vi "Forward by Address.vi"(6 "Message Priority (Normal)":T1=enum."Normal", 8 "error in (no error)":errorcluster, 9 "Message":refnum<class "Message.lvclass">, 10 "Target Enqueuer ID":string, 11 "Publisher in":refnum<class "Publisher.lvclass">) -> (0 "error out":errorcluster, 1 "Message forwarded?":bool, 3 "Publisher out":refnum<class "Publisher.lvclass">)   [LabVIEW 2020, in "Publisher.lvlib" / "Publisher.lvclass"]
doc: "Send 'Message' to the actor with 'Target Enqueuer ID'."
uses:
  Publisher.lvclass
  PPL/HDH.Actor Framework.Core.Actor.lvlibp/1abvi3w/vi.lib/ActorFramework/Message Enqueuer/Message Priority.ctl
  PPL/HDH.Actor Framework.Core.Actor.lvlibp/1abvi3w/vi.lib/ActorFramework/Message/Message.lvclass
  Publisher.lvclass/Publisher.ctl
  PPL/HDH.Actor Framework.Core.Actor.lvlibp/1abvi3w/vi.lib/ActorFramework/Message Enqueuer/Message Enqueuer.lvclass
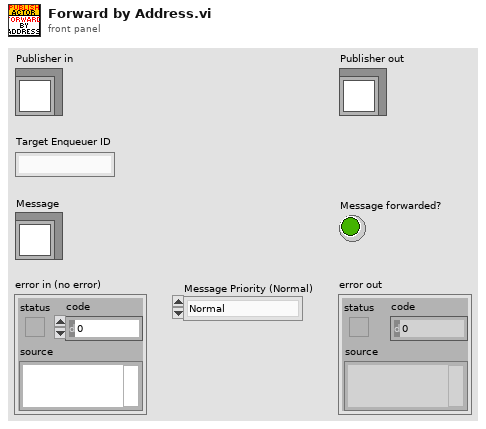
[diagram p1: front panel]
types:
  T1 = typedef "HDH.Actor Framework.Core.Actor.lvlibp/Message Enqueuer.lvclass/Message Priority.ctl" = enum16{"Low", "Normal", "High"}
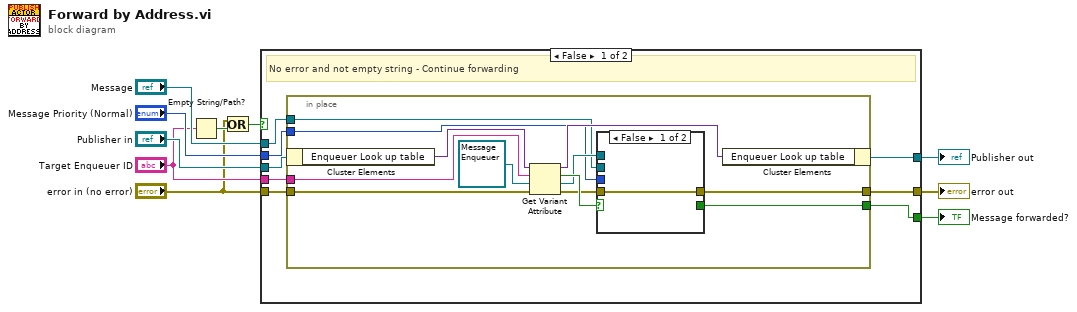
[diagram p0: block diagram]
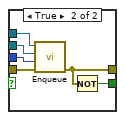
[diagram p2: hidden frame]
diagram:
  n1 = Empty String/Path?(string/path="Target Enqueuer ID") -> (empty?=w6:bool)
  n2 = Or(x="error in (no error)", y=w6) -> (x .or. y?=w5:bool)
  n3 = case shown="False" w5 {
    tunnel: [w17 w39] -> w9
    tunnel: "Publisher in" -> [w18 w39]
    tunnel: "Message" -> [w16 _]
    tunnel: "Message Priority (Normal)" -> [w15 _]
    tunnel: "Target Enqueuer ID" -> [w14 _]
    tunnel: "error in (no error)" -> [w13 w38]
    tunnel: [w11 _] -> w2
    tunnel: [w12 w38] -> w1
    frame False {
      # "No error and not empty string - Continue forwarding"
      n4 = in-place {
        in-place-border: w16 -> [w20]
        in-place-border: w15 -> [w19]
        in-place-border: w14 -> [w28]
        in-place-border: w13 -> [w26]
        in-place-border: [w24] -> w12
        in-place-border: [w22] -> w11
        n5 = in-place-cluster #1(w18) -> ("Enqueuer Look up table"=w30:variant)
        n6 = Get Variant Attribute(Variant=w30, name=w28, default value (empty Variant)=refnum<class "Message Enqueuer.lvclass"> refnum ("value"), error in=w26) -> (duplicate Variant=w29:variant, found=w25:bool, value=w21:refnum<class "Message Enqueuer.lvclass">, error out=w23:errorcluster)
        n7 = case shown="False" w25 {
          tunnel: [w31 w33] -> w24
          tunnel: w23 -> [w31 w34]
          tunnel: [_ w32] -> w22
          tunnel: w21 -> [_ w37]
          tunnel: w20 -> [_ w36]
          tunnel: w19 -> [_ w35]
          frame False {
          }
          frame True {
            n8 = call "Enqueue.vi"("error in (no error)"=w34, "Message Priority (Normal)"=w35, "Message"=w36, "Message Enqueuer in"=w37) -> ("error out"=w33:errorcluster)  [unwired: 6 in, 1 out]
            n9 = Not(x=w33) -> (.not. x?=w32:bool)
          }
        }
        n10 = in-place-cluster #1("Enqueuer Look up table"=w29) -> (w17:refnum<class "Publisher.lvclass">)
      }
    }
    frame True {
      # "Error or no target - Abort operation"
    }
  }
  "error out" <- w1
  "Publisher out" <- w9
  "Message forwarded?" <- w2
